vi "Transfer Properties to New Node.vi"(7 "Replacement Channels":T1={"Channel to Replace"="Targets/Controller/Custom Devices/VCOM/CAN_Sender_Tx/ACC/ACC_ESP_E2E_PR2/ACC_NEW_SIGNAL", "Replacement Channel"="Targets/Controller/User Channels/User Channel 1"}, 8 "error in (no error)":errorcluster, 10 "Property Type":i32(ring)=8 items=["K_STRING", "K_BOOL", "K_I32", "K_U32", "K_DOUBLE", "K_U64", "K_VARIANT", "K_DEPENDENTFILE", "K_DEPENDENTNODE", "K_DATASOURCENODE", "K_U16", "K_DBLARR", "K_U32ARR", "K_I32ARR", "K_STRINGARR", "K_DICTIONARY", "K_DICTIONARYARR", "K_BINARYSTRING", "K_I16", "K_I64", "K_BOOLARR", "K_U64ARR", "K_U16ARR", "K_I64ARR", "K_I16ARR"], 11 "reference":refnum<k24>) -> (0 "error out":errorcluster, 2 "Replacement Log":string[](array[string]), 3 "reference out":refnum<k24>)   [LabVIEW 2025]
uses:
  Controls/Replacement Channels.ctl
  NationalInstruments.VeriStand.SystemDefinitionAPI
  NationalInstruments.VeriStand.SystemStorage
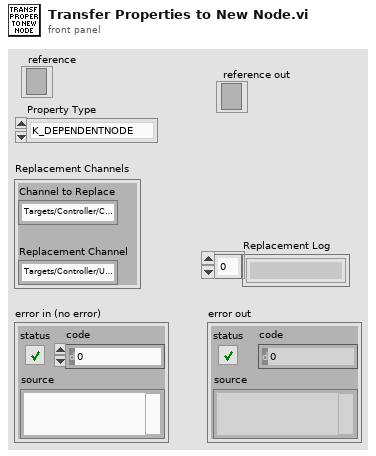
[diagram p1: front panel]
types:
  T1 = typedef "Replacement Channels.ctl" = cluster{"Channel to Replace":string, "Replacement Channel":string}
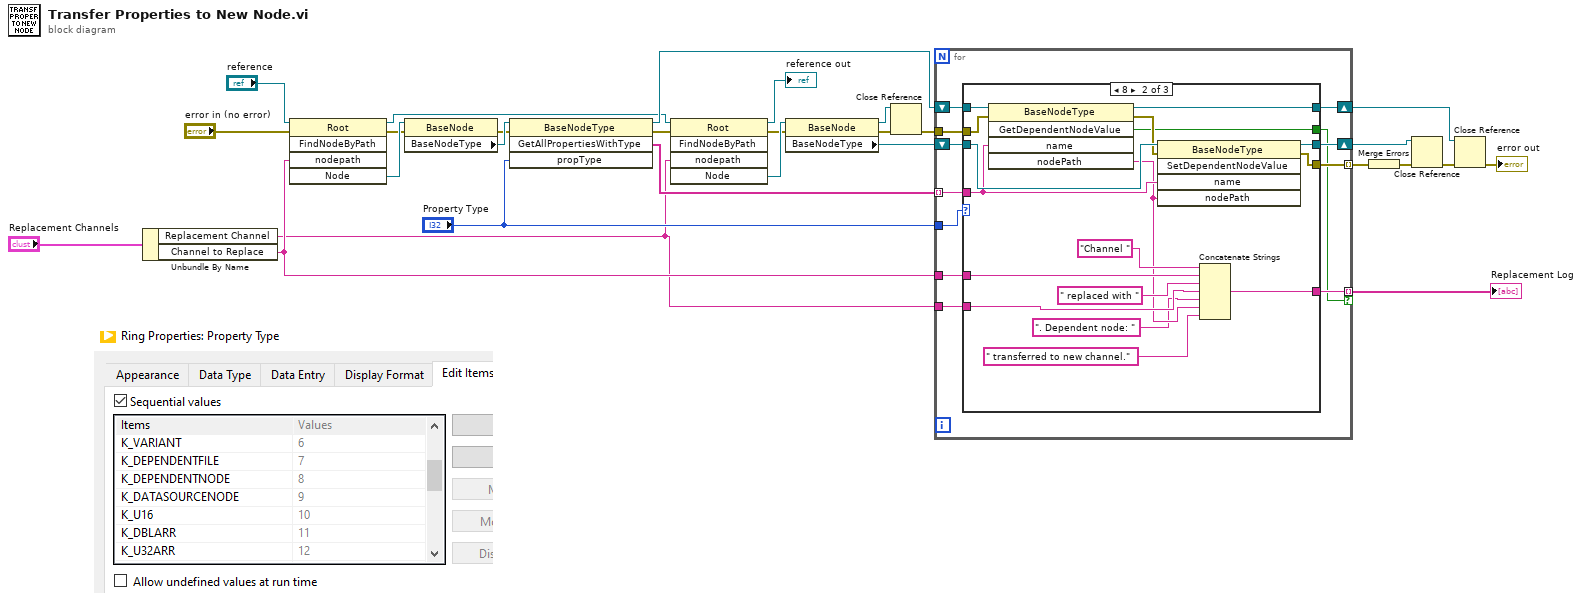
[diagram p0: block diagram]
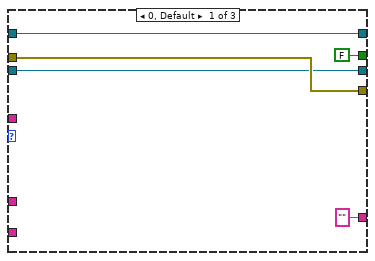
[diagram p2: hidden frame]
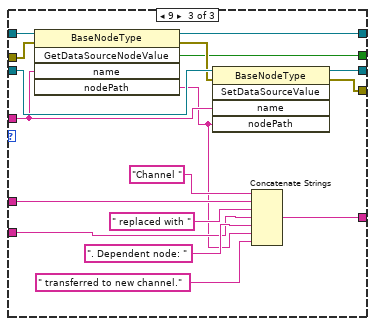
[diagram p3: hidden frame]
diagram:
  n1 = Unbundle By Name("Replacement Channels") -> ("Replacement Channel"=w2:string, "Channel to Replace"=w3:string)
  n2 = invoke class="Root" method="FindNodeByPath"(reference="reference", error in="error in (no error)", "nodepath"=w3) -> (reference out=w6:refnum<k24>, error out=w25:errorcluster, "Node"=w27:refnum<k24>)  [unwired: 2 in, 2 out]
  n3 = property class="BaseNode"(reference=w27, error in=w25) -> (error out=w24:errorcluster, "BaseNodeType"=w26:refnum<k24>)  [unwired: 1 out]
  n4 = invoke class="BaseNodeType" method="GetAllPropertiesWithType"(reference=w26, error in=w24, "propType"="Property Type") -> (reference out=w18:refnum<k24>, error out=w22:errorcluster, "GetAllPropertiesWithType"=w20:string[])  [unwired: 1 in, 1 out]
  n5 = invoke class="Root" method="FindNodeByPath"(reference=w6, error in=w22, "nodepath"=w2) -> (reference out=→"reference out":refnum<k24>, error out=w16:errorcluster, "Node"=w23:refnum<k24>)  [unwired: 2 in, 2 out]
  n6 = property class="BaseNode"(reference=w23, error in=w16) -> (reference out=w14:refnum<k24>, error out=w15:errorcluster, "BaseNodeType"=w21:refnum<k24>)
  n7 = Close Reference(reference=w14, error in (no error)=w15) -> (error out=w13:errorcluster)
  n8 = for {
    tunnel: w13 -> [w39]
    tunnel: w20 -> [w38] mode=indexing
    tunnel: [w37] -> w19 mode=indexing
    tunnel: "Property Type" -> [w35]
    shift-right: [w34] -> w11
    shift-left: w21 -> [w40]
    shift-right: [w33] -> w9
    shift-left: w18 -> [w36]
    tunnel: w3 -> [w32]
    tunnel: w2 -> [w31]
    tunnel: [w30] -> w1 mode=indexing if=w29
    n9 = case shown="8" w35 {
      tunnel: w40 -> [w44 w62 w79]
      tunnel: w39 -> [w45 w61 w78]
      tunnel: w38 -> [_ w59 w76]
      tunnel: [w45 w58 w75] -> w37
      tunnel: w36 -> [w43 w57 w74]
      tunnel: [w44 w56 w73] -> w34
      tunnel: [w43 w55 w72] -> w33
      tunnel: w32 -> [_ w52 w67]
      tunnel: w31 -> [_ w51 w66]
      tunnel: ["" w47 w64] -> w30
      tunnel: [FALSE ("GetDataSourceNodeValue") w46 w63] -> w29
      frame 0, Default {
      }
      frame 8 {
        n10 = invoke class="BaseNodeType" method="GetDependentNodeValue"(reference=w57, error in=w61, "name"=w59) -> (reference out=w55:refnum<k24>, error out=w60:errorcluster, "GetDependentNodeValue"=w46:bool, "nodePath"=w50:string)  [unwired: 2 in, 1 out]
        n11 = invoke class="BaseNodeType" method="SetDependentNodeValue"(reference=w62, error in=w60, "name"=w59, "nodePath"=w50) -> (reference out=w56:refnum<k24>, error out=w58:errorcluster)  [unwired: 1 in, 3 out]
        n12 = Concatenate Strings("Channel " ("string"), w52, " replaced with " ("string"), w51, ". Dependent node: " ("string"), w50, " transferred to new channel." ("string")) -> (w47:string)
      }
      frame 9 {
        n13 = invoke class="BaseNodeType" method="GetDataSourceNodeValue"(reference=w74, error in=w78, "name"=w76) -> (reference out=w72:refnum<k24>, error out=w77:errorcluster, "GetDataSourceNodeValue"=w63:bool, "nodePath"=w65:string)  [unwired: 2 in, 1 out]
        n14 = invoke class="BaseNodeType" method="SetDataSourceValue"(reference=w79, error in=w77, "name"=w76, "nodePath"=w65) -> (reference out=w73:refnum<k24>, error out=w75:errorcluster)  [unwired: 1 in, 3 out]
        n15 = Concatenate Strings("Channel " ("string"), w67, " replaced with " ("string"), w66, ". Dependent node: " ("string"), w65, " transferred to new channel." ("string")) -> (w64:string)
      }
    }
  }
  "Replacement Log" <- w1
  n16 = Merge Errors(w19) -> (w12:errorcluster)
  n17 = Close Reference(reference=w11, error in (no error)=w12) -> (error out=w10:errorcluster)
  n18 = Close Reference(reference=w9, error in (no error)=w10) -> (error out=→"error out":errorcluster)
